vi "ExtractMeasurementDataFromCOMbuffer.vi"(8 "error in (no error)":errorcluster, 11 "Input OPC data":string) -> (0 "error out":errorcluster, 1 "Output Number of Particles per 100 CC":i32[](array[numeric]), 2 "Valid Data":bool, 3 "Output OPC data":string)   [LabVIEW 2013]
doc: "Use this template to build a VI to use as a subVI."
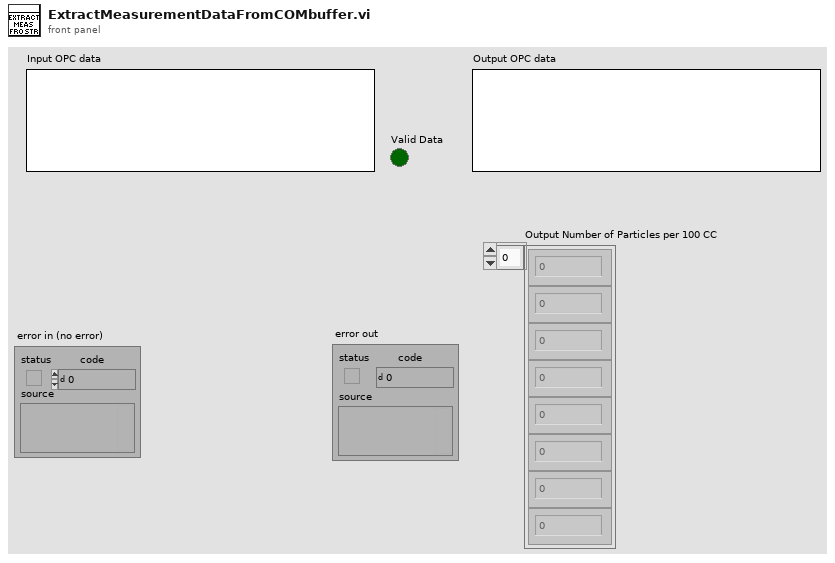
[diagram p1: front panel]
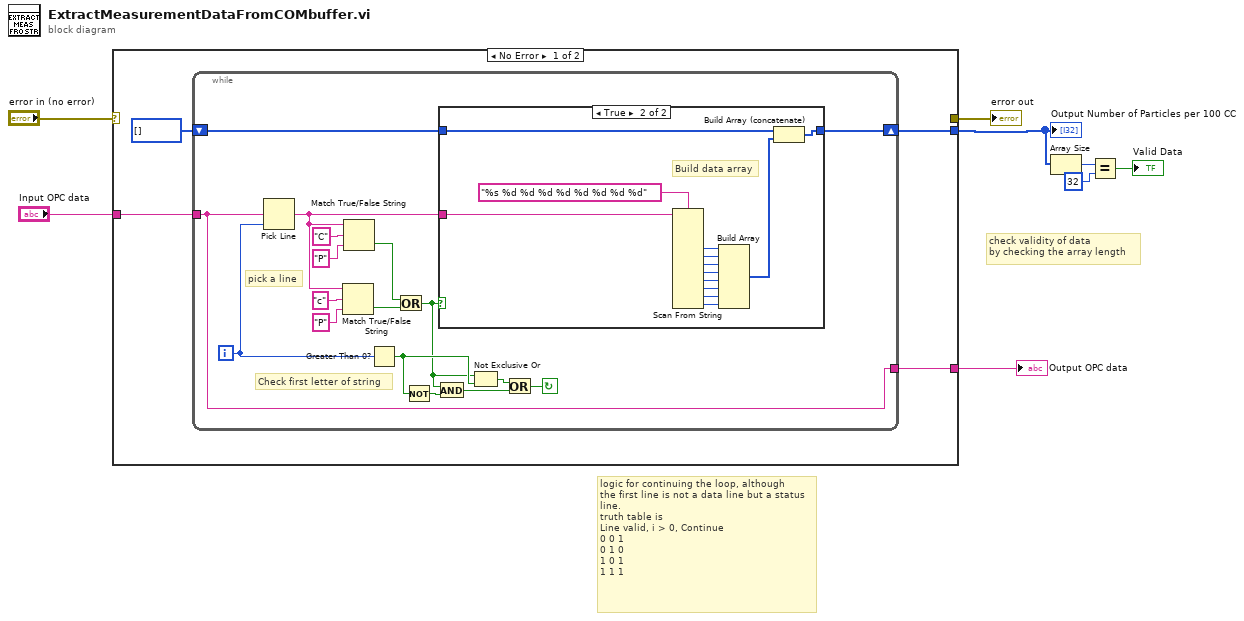
[diagram p0: block diagram]
diagram:
  # "logic for continuing the loop, although\nthe first line is not a data line but a status\nline.\ntruth table is \nLine valid, i > 0, Continue\n0 0 1\n0 1 0\n1 0 1\n1 1 1"
  # "check validity of data\nby checking the array length"
  n1 = case shown="No Error" "error in (no error)" {
    selector: "error in (no error)" -> [_ w44]
    tunnel: [_ w44] -> w7
    tunnel: "Input OPC data" -> [w12 _]
    tunnel: [w10 _] -> w5
    tunnel: [w9 _] -> w1
    frame No Error {
      n2 = while {
        tunnel: w12 -> [w13]
        shift-right: [w21] -> w10
        shift-left: i32[] [] ("Output Number of Particles per 100 CC") -> [w22]
        tunnel: [w13] -> w9
        i -> [w20]
        stop <- w14 continue-if-true
        # "pick a line"
        # "Check first letter of string"
        n3 = Pick Line(multi-line string=w13, line index=w20) -> (output string=w23:string)  [unwired: 1 in]
        n4 = Match True/False String(2:"P" ("false string"), 3:"c" ("true string"), 4:w23) -> (0:w29:bool)  [unwired: 1 out]
        n5 = Match True/False String(2:"P" ("false string"), 3:"C" ("true string"), 4:w23) -> (0:w26:bool)  [unwired: 1 out]
        n6 = Greater Than 0?(x=w20) -> (x > 0?=w18:bool)
        n7 = Or(x=w26, y=w29) -> (x .or. y?=w17:bool)
        n8 = Not(x=w18) -> (.not. x?=w19:bool)
        n9 = And(x=w17, y=w19) -> (x .and. y?=w15:bool)
        n10 = case shown="True" w17 {
          tunnel: w23 -> [_ w35]
          tunnel: w22 -> [w30 w33]
          tunnel: [w30 w31] -> w21
          frame False {
          }
          frame True {
            # "Build data array"
            n11 = Scan From String(format string="%s %d %d %d %d %d %d %d %d", input string=w35) -> (output 2=w36:i32, output 3=w37:i32, output 4=w38:i32, output 5=w39:i32, output 6=w40:i32, output 7=w41:i32, output 8=w42:i32, output 9=w43:i32)  [unwired: 12 in, 3 out]
            n12 = Build Array(w36, w37, w38, w39, w40, w41, w42, w43) -> (w32:i32[])
            n13 = Build Array (concatenate)(w33, w32) -> (w31:i32[])
          }
        }
        n14 = Not Exclusive Or(1:w18, 2:w17) -> (0:w16:bool)
        n15 = Or(x=w16, y=w15) -> (x .or. y?=w14:bool)
      }
    }
    frame Error {
    }
  }
  "error out" <- w7
  "Output Number of Particles per 100 CC" <- w5
  "Output OPC data" <- w1
  n16 = Array Size(array=w5) -> (size(s)=w4:i32)
  n17 = Equal?(x=w4, y=32) -> (x = y?=→"Valid Data":bool)
